vi "Client.vi"() -> ()   [LabVIEW 2020]
panel:
  in  "Tab Control":T1(tab)
  in  "Balcony Temperature Control":dbl
  in  "Bedroom 2 Temperature Control":dbl
  in  "Bedroom 1 Temperature Control":dbl
  in  "Kitchen Temperature Control":dbl
  in  "Master Bedroom Temperature Control":dbl
  in  "Time Control":dbl(knob) scale=0.0..24.0
  in  "Living Room Temperature Control":dbl
  in  "Light Rotation":bool
  in  "Balcony Alarm":bool
  in  "Bedroom 2 Alarm":bool
  in  "Bedroom 1 Alarm":bool
  in  "Kitchen Alarm":bool
  in  "Master Bedroom Alarm":bool
  in  "Automatic Curtain":bool
  in  "Living Room Alarm":bool
  in  "Curtains Master Button":bool
  in  "Doors Master Button":bool
  in  "Lights Master Button":bool
  in  "TV Brightness":dbl(knob) scale=1.0..6.0
  in  "Adaptive Brightness":bool
  in  "TV Volume":i32(knob) scale=0.0..100.0
  in  "TV Fast Forward Reverse":bool
  in  "TV Fast Forward":bool
  in  "TV Channel 2":bool
  in  "TV Channel 1":bool
  in  "TV Pause":bool
  in  "TV Play":bool
  in  "TV On/Off":bool
  in  "Living Room Curtain":bool
  in  "Living Room Light 1":bool
  in  "Living Room Light 2":bool
  in  "Living Room Light 1 Dim":bool
  in  "Living Room Light 2 Dim":bool
  in  "Living Room Door":bool
  in  "Master Bedroom AC":bool
  in  "Master Bedroom Curtain":bool
  in  "Master Bedroom Door":bool
  in  "Master Bedroom Light 2 Dim":bool
  in  "Master Bedroom Light 1 Dim":bool
  in  "Master Bedroom Light 2":bool
  in  "Master Bedroom Light 1":bool
  in  "Bedroom 1 Door":bool
  in  "Bedroom 1 Curtain":bool
  in  "Bedroom 1 Light 1 Dim":bool
  in  "Bedroom 1 Light 1":bool
  in  "Bedroom 2 Door":bool
  in  "Bedroom 2 Curtain":bool
  in  "Bedroom 2 Light 1 Dim":bool
  in  "Bedroom 2 Light 1":bool
  in  "Balcony Door 2":bool
  in  "Balcony Door 1":bool
  in  "Balcony Light 3 Dim":bool
  in  "Balcony Light 2 Dim":bool
  in  "Balcony Light 1 Dim":bool
  in  "Balcony Light 3":bool
  in  "Balcony Light 2":bool
  in  "Balcony Light 1":bool
  in  "Kitchen Door 2":bool
  in  "Kitchen Door 1":bool
  in  "Kitchen Light 1 Dim":bool
  in  "Kitchen Light 1":bool
  in  "stop":bool
  # "CLIENT"
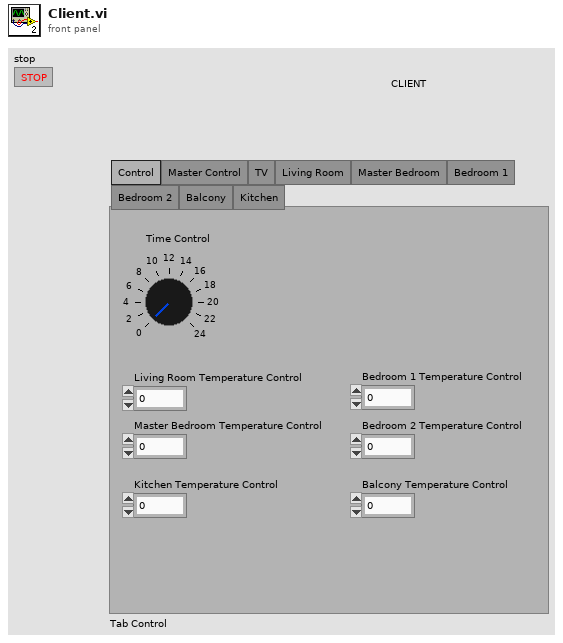
[diagram p1: front panel]
types:
  T1 = enum32{"Control", "Master Control", "TV", "Living Room", "Master Bedroom", "Bedroom 1", "Bedroom 2", "Balcony", "Kitchen"}
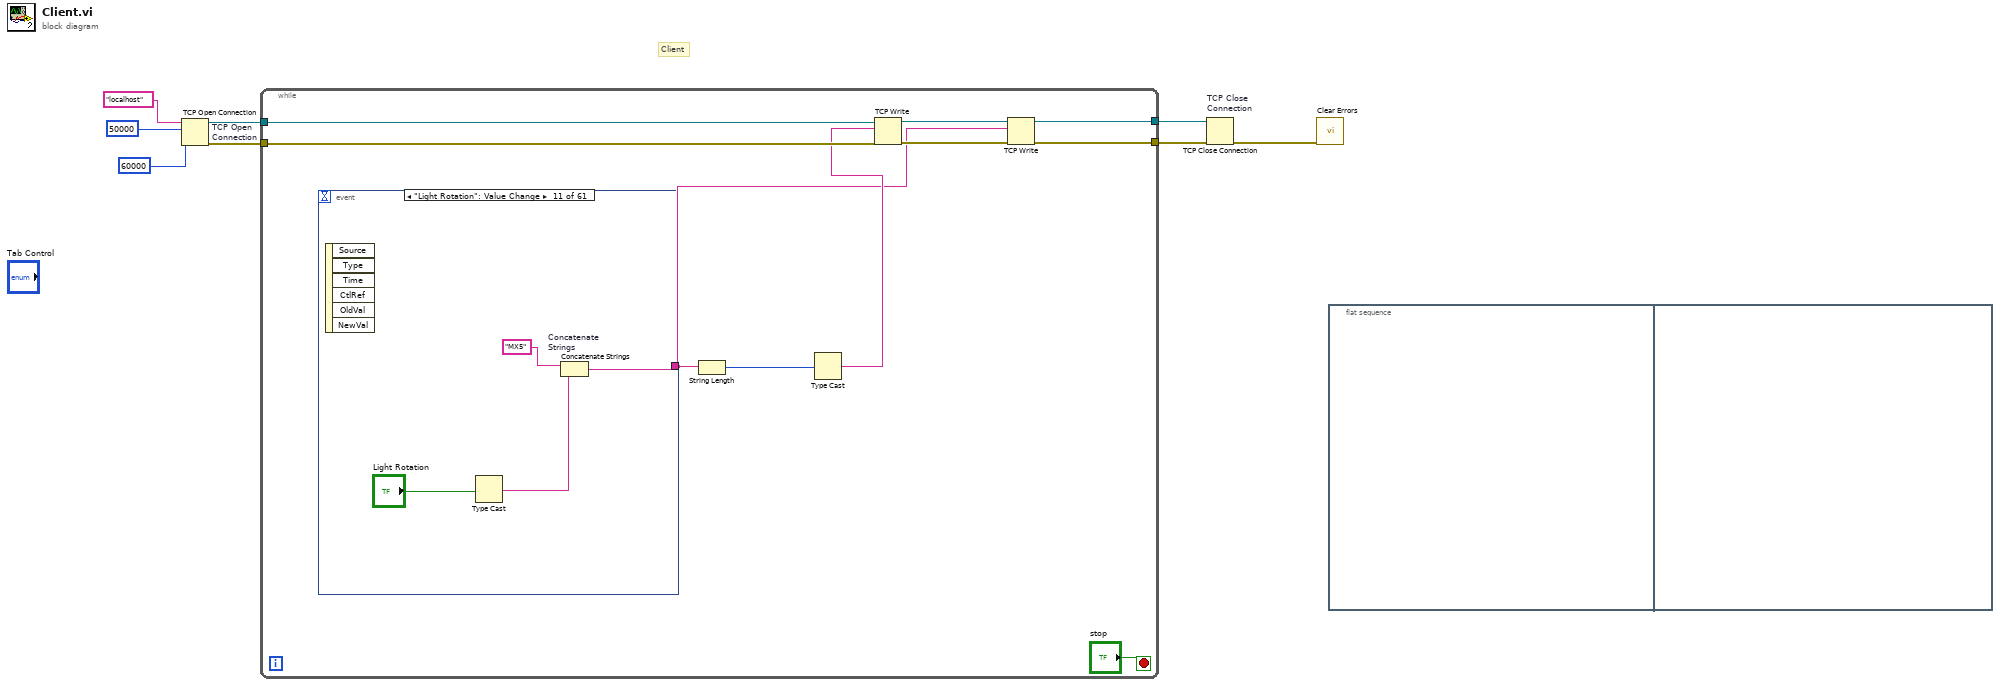
[diagram p0: block diagram]
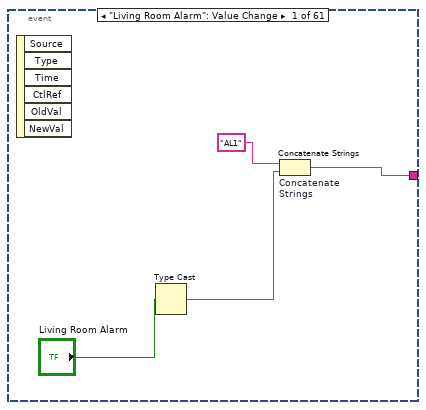
[diagram p2: hidden frame]
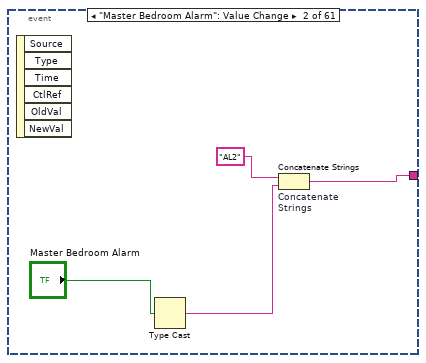
[diagram p3: hidden frame]
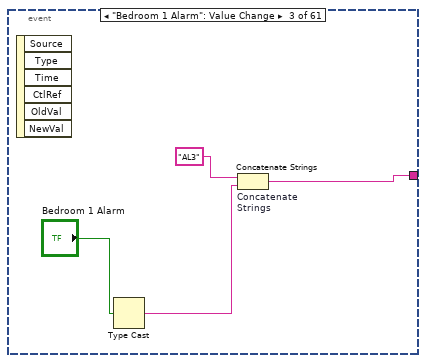
[diagram p4: hidden frame]
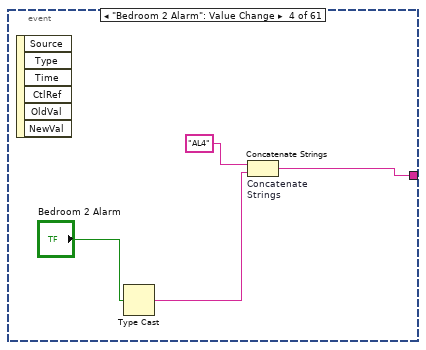
[diagram p5: hidden frame]
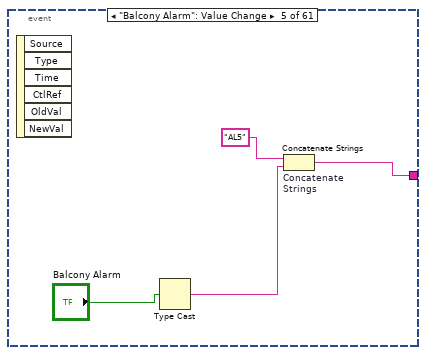
[diagram p6: hidden frame]
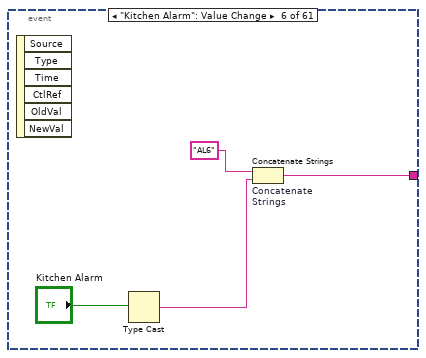
[diagram p7: hidden frame]
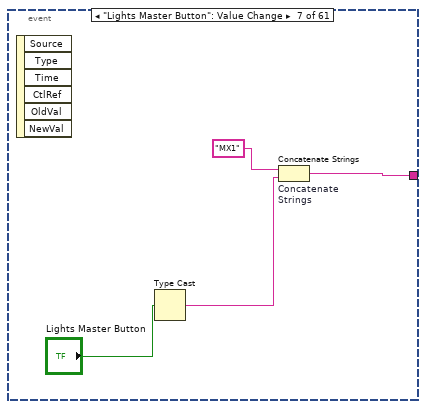
[diagram p8: hidden frame]
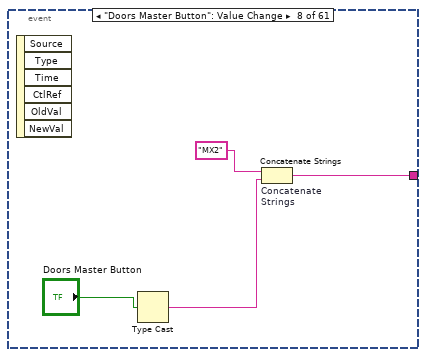
[diagram p9: hidden frame]
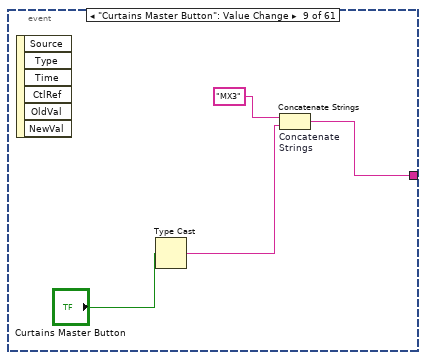
[diagram p10: hidden frame]
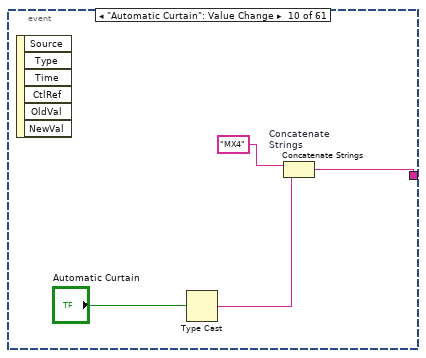
[diagram p11: hidden frame]
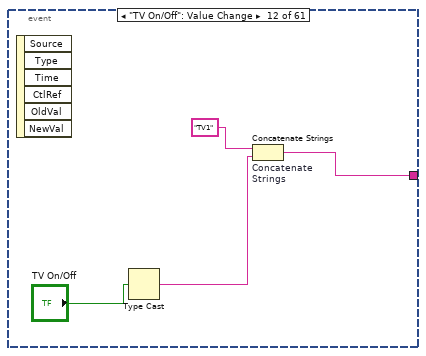
[diagram p12: hidden frame]
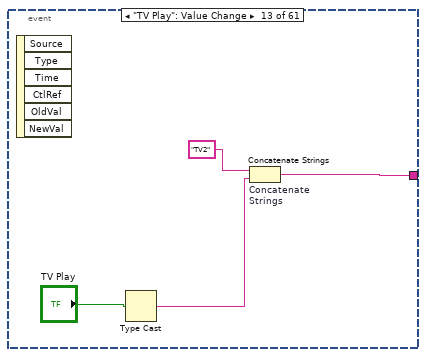
[diagram p13: hidden frame]
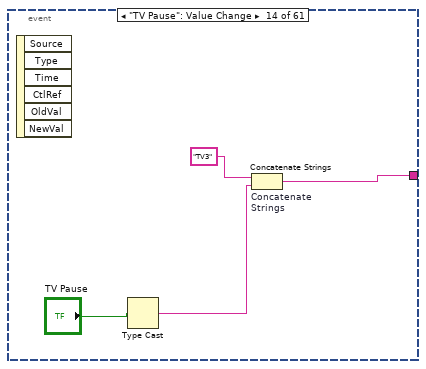
[diagram p14: hidden frame]
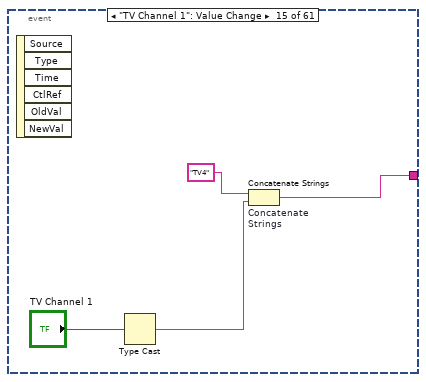
[diagram p15: hidden frame]
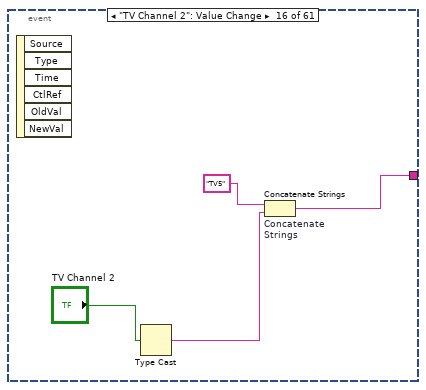
[diagram p16: hidden frame]
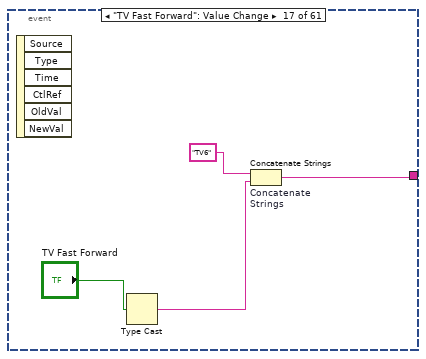
[diagram p17: hidden frame]
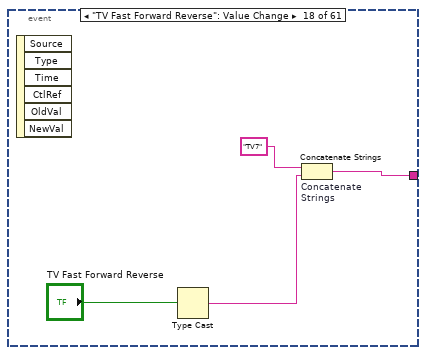
[diagram p18: hidden frame]
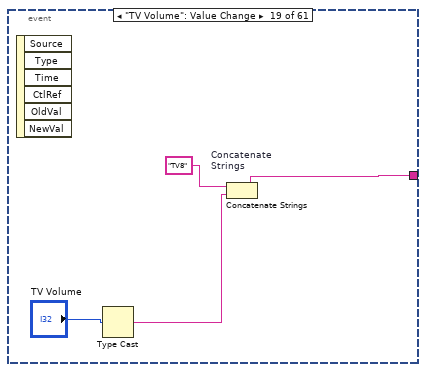
[diagram p19: hidden frame]
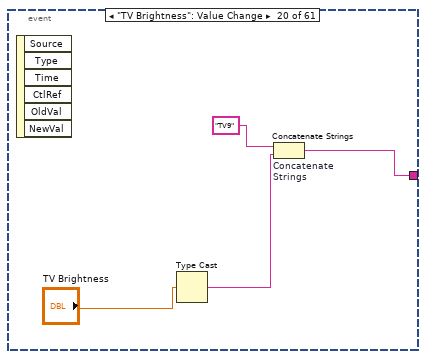
[diagram p20: hidden frame]
diagram:
  # "Client"
  n1 = TCP Open Connection "TCP Open \nConnection"(address="localhost", remote port or service name=u16 50000, timeout ms (60000)=60000) -> (connection ID=w5:refnum<k5>, error out=w3:errorcluster)  [unwired: 2 in]
  n2 = while {
    tunnel: w5 -> [w17]
    tunnel: [w15] -> w4
    tunnel: w3 -> [w14]
    tunnel: [w12] -> w2
    stop <- "stop" stop-if-true
    n3 = event shown="[10] \"Light Rotation\": Value Change" {
      selector: _ -> [_ _ _ _ _ _ _ _ _ _ _ _ _ _ _ _ _ _ _ _ _ _ _ _ _ _ _ _ _ _ _ _ _ _ _ _ _ _ _ _ _ _ _ _ _ _ _ _ _ _ _ _ _ _ _ _ _ _ _ _ _]
      dyn-events: _ -> [_ _ _ _ _ _ _ _ _ _ _ _ _ _ _ _ _ _ _ _ _ _ _ _ _ _ _ _ _ _ _ _ _ _ _ _ _ _ _ _ _ _ _ _ _ _ _ _ _ _ _ _ _ _ _ _ _ _ _ _ _]
      timeout: _ -> [_ _ _ _ _ _ _ _ _ _ _ _ _ _ _ _ _ _ _ _ _ _ _ _ _ _ _ _ _ _ _ _ _ _ _ _ _ _ _ _ _ _ _ _ _ _ _ _ _ _ _ _ _ _ _ _ _ _ _ _ _]
      tunnel: [w20 w24 w28 w32 w36 w40 w43 w48 w51 w55 w60 w63 w68 w72 w75 w80 w84 w87 w91 w96 w99 w105 w108 w112 w116 w120 w124 w127 w131 w136 w139 w144 w148 w152 w155 w160 w163 w168 w171 w176 w180 w183 w188 w192 w195 w199 w203 w208 w212 w216 w220 w224 w228 w232 w236 w240 w244 w248 w252 w256 w260] -> w9
      event "Living Room Alarm": Value Change {
        n4 = event-data() -> ()  [unwired: 1 in, 6 out]
        n5 = Type Cast(x="Living Room Alarm") -> (*(type *) &x=w22:string)  [unwired: 1 in]
        n6 = Concatenate Strings "Concatenate \nStrings"("AL1" ("string"), w22) -> (w20:string)
      }
      event "Master Bedroom Alarm": Value Change {
        n7 = event-data() -> ()  [unwired: 1 in, 6 out]
        n8 = Type Cast(x="Master Bedroom Alarm") -> (*(type *) &x=w26:string)  [unwired: 1 in]
        n9 = Concatenate Strings "Concatenate \nStrings"("AL2" ("string"), w26) -> (w24:string)
      }
      event "Bedroom 1 Alarm": Value Change {
        n10 = event-data() -> ()  [unwired: 1 in, 6 out]
        n11 = Type Cast(x="Bedroom 1 Alarm") -> (*(type *) &x=w30:string)  [unwired: 1 in]
        n12 = Concatenate Strings "Concatenate \nStrings"("AL3" ("string"), w30) -> (w28:string)
      }
      event "Bedroom 2 Alarm": Value Change {
        n13 = event-data() -> ()  [unwired: 1 in, 6 out]
        n14 = Type Cast(x="Bedroom 2 Alarm") -> (*(type *) &x=w34:string)  [unwired: 1 in]
        n15 = Concatenate Strings "Concatenate \nStrings"("AL4" ("string"), w34) -> (w32:string)
      }
      event "Balcony Alarm": Value Change {
        n16 = event-data() -> ()  [unwired: 1 in, 6 out]
        n17 = Type Cast(x="Balcony Alarm") -> (*(type *) &x=w38:string)  [unwired: 1 in]
        n18 = Concatenate Strings "Concatenate \nStrings"("AL5" ("string"), w38) -> (w36:string)
      }
      event "Kitchen Alarm": Value Change {
        n19 = event-data() -> ()  [unwired: 1 in, 6 out]
        n20 = Type Cast(x="Kitchen Alarm") -> (*(type *) &x=w42:string)  [unwired: 1 in]
        n21 = Concatenate Strings "Concatenate \nStrings"("AL6" ("string"), w42) -> (w40:string)
      }
      event "Lights Master Button": Value Change {
        n22 = event-data() -> ()  [unwired: 1 in, 6 out]
        n23 = Type Cast(x="Lights Master Button") -> (*(type *) &x=w45:string)  [unwired: 1 in]
        n24 = Concatenate Strings "Concatenate \nStrings"("MX1" ("string"), w45) -> (w43:string)
      }
      event "Doors Master Button": Value Change {
        n25 = event-data() -> ()  [unwired: 1 in, 6 out]
        n26 = Type Cast(x="Doors Master Button") -> (*(type *) &x=w50:string)  [unwired: 1 in]
        n27 = Concatenate Strings "Concatenate \nStrings"("MX2" ("string"), w50) -> (w48:string)
      }
      event "Curtains Master Button": Value Change {
        n28 = event-data() -> ()  [unwired: 1 in, 6 out]
        n29 = Type Cast(x="Curtains Master Button") -> (*(type *) &x=w54:string)  [unwired: 1 in]
        n30 = Concatenate Strings "Concatenate \nStrings"("MX3" ("string"), w54) -> (w51:string)
      }
      event "Automatic Curtain": Value Change {
        n31 = event-data() -> ()  [unwired: 1 in, 6 out]
        n32 = Type Cast(x="Automatic Curtain") -> (*(type *) &x=w57:string)  [unwired: 1 in]
        n33 = Concatenate Strings "Concatenate \nStrings"("MX4" ("string"), w57) -> (w55:string)
      }
      event "Light Rotation": Value Change {
        n34 = event-data() -> ()  [unwired: 1 in, 6 out]
        n35 = Type Cast(x="Light Rotation") -> (*(type *) &x=w62:string)  [unwired: 1 in]
        n36 = Concatenate Strings "Concatenate \nStrings"("MX5" ("string"), w62) -> (w60:string)
      }
      event "TV On/Off": Value Change {
        n37 = event-data() -> ()  [unwired: 1 in, 6 out]
        n38 = Type Cast(x="TV On/Off") -> (*(type *) &x=w66:string)  [unwired: 1 in]
        n39 = Concatenate Strings "Concatenate \nStrings"("TV1" ("string"), w66) -> (w63:string)
      }
      event "TV Play": Value Change {
        n40 = event-data() -> ()  [unwired: 1 in, 6 out]
        n41 = Type Cast(x="TV Play") -> (*(type *) &x=w70:string)  [unwired: 1 in]
        n42 = Concatenate Strings "Concatenate \nStrings"("TV2" ("string"), w70) -> (w68:string)
      }
      event "TV Pause": Value Change {
        n43 = event-data() -> ()  [unwired: 1 in, 6 out]
        n44 = Type Cast(x="TV Pause") -> (*(type *) &x=w74:string)  [unwired: 1 in]
        n45 = Concatenate Strings "Concatenate \nStrings"("TV3" ("string"), w74) -> (w72:string)
      }
      event "TV Channel 1": Value Change {
        n46 = event-data() -> ()  [unwired: 1 in, 6 out]
        n47 = Type Cast(x="TV Channel 1") -> (*(type *) &x=w78:string)  [unwired: 1 in]
        n48 = Concatenate Strings "Concatenate \nStrings"("TV4" ("string"), w78) -> (w75:string)
      }
      event "TV Channel 2": Value Change {
        n49 = event-data() -> ()  [unwired: 1 in, 6 out]
        n50 = Type Cast(x="TV Channel 2") -> (*(type *) &x=w82:string)  [unwired: 1 in]
        n51 = Concatenate Strings "Concatenate \nStrings"("TV5" ("string"), w82) -> (w80:string)
      }
      event "TV Fast Forward": Value Change {
        n52 = event-data() -> ()  [unwired: 1 in, 6 out]
        n53 = Type Cast(x="TV Fast Forward") -> (*(type *) &x=w86:string)  [unwired: 1 in]
        n54 = Concatenate Strings "Concatenate \nStrings"("TV6" ("string"), w86) -> (w84:string)
      }
      event "TV Fast Forward Reverse": Value Change {
        n55 = event-data() -> ()  [unwired: 1 in, 6 out]
        n56 = Type Cast(x="TV Fast Forward Reverse") -> (*(type *) &x=w90:string)  [unwired: 1 in]
        n57 = Concatenate Strings "Concatenate \nStrings"("TV7" ("string"), w90) -> (w87:string)
      }
      event "TV Volume": Value Change {
        n58 = event-data() -> ()  [unwired: 1 in, 6 out]
        n59 = Type Cast(x="TV Volume") -> (*(type *) &x=w94:string)  [unwired: 1 in]
        n60 = Concatenate Strings "Concatenate \nStrings"("TV8" ("string"), w94) -> (w91:string)
      }
      event "TV Brightness": Value Change {
        n61 = event-data() -> ()  [unwired: 1 in, 6 out]
        n62 = Type Cast(x="TV Brightness") -> (*(type *) &x=w98:string)  [unwired: 1 in]
        n63 = Concatenate Strings "Concatenate \nStrings"("TV9" ("string"), w98) -> (w96:string)
      }
      event "Adaptive Brightness": Value Change {
        n64 = event-data() -> ()  [unwired: 1 in, 6 out]
        n65 = Type Cast(x="Adaptive Brightness") -> (*(type *) &x=w102:string)  [unwired: 1 in]
        n66 = Concatenate Strings "Concatenate \nStrings"("TV10" ("string"), w102) -> (w99:string)
      }
      event "Living Room Temperature Control": Value Change {
        n67 = event-data() -> ()  [unwired: 1 in, 6 out]
        n68 = Type Cast(x="Living Room Temperature Control") -> (*(type *) &x=w104:string)  [unwired: 1 in]
        n69 = Concatenate Strings "Concatenate \nStrings"("HX1" ("string"), w104) -> (w105:string)
      }
      event "Master Bedroom Temperature Control": Value Change {
        n70 = event-data() -> ()  [unwired: 1 in, 6 out]
        n71 = Type Cast(x="Master Bedroom Temperature Control") -> (*(type *) &x=w110:string)  [unwired: 1 in]
        n72 = Concatenate Strings "Concatenate \nStrings"("HX3" ("string"), w110) -> (w108:string)
      }
      event "Bedroom 1 Temperature Control": Value Change {
        n73 = event-data() -> ()  [unwired: 1 in, 6 out]
        n74 = Type Cast(x="Bedroom 1 Temperature Control") -> (*(type *) &x=w113:string)  [unwired: 1 in]
        n75 = Concatenate Strings "Concatenate \nStrings"("HX4" ("string"), w113) -> (w112:string)
      }
      event "Bedroom 2 Temperature Control": Value Change {
        n76 = event-data() -> ()  [unwired: 1 in, 6 out]
        n77 = Type Cast(x="Bedroom 2 Temperature Control") -> (*(type *) &x=w118:string)  [unwired: 1 in]
        n78 = Concatenate Strings "Concatenate \nStrings"("HX5" ("string"), w118) -> (w116:string)
      }
      event "Balcony Temperature Control": Value Change {
        n79 = event-data() -> ()  [unwired: 1 in, 6 out]
        n80 = Type Cast(x="Balcony Temperature Control") -> (*(type *) &x=w122:string)  [unwired: 1 in]
        n81 = Concatenate Strings "Concatenate \nStrings"("HX6" ("string"), w122) -> (w120:string)
      }
      event "Kitchen Temperature Control": Value Change {
        n82 = event-data() -> ()  [unwired: 1 in, 6 out]
        n83 = Type Cast(x="Kitchen Temperature Control") -> (*(type *) &x=w125:string)  [unwired: 1 in]
        n84 = Concatenate Strings "Concatenate \nStrings"("HX7" ("string"), w125) -> (w124:string)
      }
      event "Time Control": Value Change {
        n85 = event-data() -> ()  [unwired: 1 in, 6 out]
        n86 = Type Cast(x="Time Control") -> (*(type *) &x=w129:string)  [unwired: 1 in]
        n87 = Concatenate Strings "Concatenate \nStrings"("HX2" ("string"), w129) -> (w127:string)
      }
      event "Living Room Light 1": Value Change {
        n88 = event-data() -> ()  [unwired: 1 in, 6 out]
        n89 = Type Cast(x="Living Room Light 1") -> (*(type *) &x=w134:string)  [unwired: 1 in]
        n90 = Concatenate Strings "Concatenate \nStrings"("LR1" ("string"), w134) -> (w131:string)
      }
      event "Living Room Light 2": Value Change {
        n91 = event-data() -> ()  [unwired: 1 in, 6 out]
        n92 = Type Cast(x="Living Room Light 2") -> (*(type *) &x=w138:string)  [unwired: 1 in]
        n93 = Concatenate Strings "Concatenate \nStrings"("LR2" ("string"), w138) -> (w136:string)
      }
      event "Living Room Light 1 Dim": Value Change {
        n94 = event-data() -> ()  [unwired: 1 in, 6 out]
        n95 = Type Cast(x="Living Room Light 1 Dim") -> (*(type *) &x=w142:string)  [unwired: 1 in]
        n96 = Concatenate Strings "Concatenate \nStrings"("LR3" ("string"), w142) -> (w139:string)
      }
      event "Living Room Light 2 Dim": Value Change {
        n97 = event-data() -> ()  [unwired: 1 in, 6 out]
        n98 = Type Cast(x="Living Room Light 2 Dim") -> (*(type *) &x=w146:string)  [unwired: 1 in]
        n99 = Concatenate Strings "Concatenate \nStrings"("LR4" ("string"), w146) -> (w144:string)
      }
      event "Living Room Curtain": Value Change {
        n100 = event-data() -> ()  [unwired: 1 in, 6 out]
        n101 = Type Cast(x="Living Room Curtain") -> (*(type *) &x=w150:string)  [unwired: 1 in]
        n102 = Concatenate Strings "Concatenate \nStrings"("LR5" ("string"), w150) -> (w148:string)
      }
      event "Living Room Door": Value Change {
        n103 = event-data() -> ()  [unwired: 1 in, 6 out]
        n104 = Type Cast(x="Living Room Door") -> (*(type *) &x=w154:string)  [unwired: 1 in]
        n105 = Concatenate Strings "Concatenate \nStrings"("LR6" ("string"), w154) -> (w152:string)
      }
      event "Master Bedroom Light 1": Value Change {
        n106 = event-data() -> ()  [unwired: 1 in, 6 out]
        n107 = Type Cast(x="Master Bedroom Light 1") -> (*(type *) &x=w158:string)  [unwired: 1 in]
        n108 = Concatenate Strings "Concatenate \nStrings"("MB1" ("string"), w158) -> (w155:string)
      }
      event "Master Bedroom Light 2": Value Change {
        n109 = event-data() -> ()  [unwired: 1 in, 6 out]
        n110 = Type Cast(x="Master Bedroom Light 2") -> (*(type *) &x=w162:string)  [unwired: 1 in]
        n111 = Concatenate Strings "Concatenate \nStrings"("MB2" ("string"), w162) -> (w160:string)
      }
      event "Master Bedroom Light 1 Dim": Value Change {
        n112 = event-data() -> ()  [unwired: 1 in, 6 out]
        n113 = Type Cast(x="Master Bedroom Light 1 Dim") -> (*(type *) &x=w166:string)  [unwired: 1 in]
        n114 = Concatenate Strings "Concatenate \nStrings"("MB3" ("string"), w166) -> (w163:string)
      }
      event "Master Bedroom Light 2 Dim": Value Change {
        n115 = event-data() -> ()  [unwired: 1 in, 6 out]
        n116 = Type Cast(x="Master Bedroom Light 2 Dim") -> (*(type *) &x=w170:string)  [unwired: 1 in]
        n117 = Concatenate Strings "Concatenate \nStrings"("MB4" ("string"), w170) -> (w168:string)
      }
      event "Master Bedroom Curtain": Value Change {
        n118 = event-data() -> ()  [unwired: 1 in, 6 out]
        n119 = Type Cast(x="Master Bedroom Curtain") -> (*(type *) &x=w174:string)  [unwired: 1 in]
        n120 = Concatenate Strings "Concatenate \nStrings"("MB5" ("string"), w174) -> (w171:string)
      }
      event "Master Bedroom Door": Value Change {
        n121 = event-data() -> ()  [unwired: 1 in, 6 out]
        n122 = Type Cast(x="Master Bedroom Door") -> (*(type *) &x=w178:string)  [unwired: 1 in]
        n123 = Concatenate Strings "Concatenate \nStrings"("MB6" ("string"), w178) -> (w176:string)
      }
      event "Master Bedroom AC": Value Change {
        n124 = event-data() -> ()  [unwired: 1 in, 6 out]
        n125 = Type Cast(x="Master Bedroom AC") -> (*(type *) &x=w182:string)  [unwired: 1 in]
        n126 = Concatenate Strings "Concatenate \nStrings"("MB7" ("string"), w182) -> (w180:string)
      }
      event "Bedroom 1 Light 1": Value Change {
        n127 = event-data() -> ()  [unwired: 1 in, 6 out]
        n128 = Type Cast(x="Bedroom 1 Light 1") -> (*(type *) &x=w186:string)  [unwired: 1 in]
        n129 = Concatenate Strings "Concatenate \nStrings"("B11" ("string"), w186) -> (w183:string)
      }
      event "Bedroom 1 Light 1 Dim": Value Change {
        n130 = event-data() -> ()  [unwired: 1 in, 6 out]
        n131 = Type Cast(x="Bedroom 1 Light 1 Dim") -> (*(type *) &x=w190:string)  [unwired: 1 in]
        n132 = Concatenate Strings "Concatenate \nStrings"("B12" ("string"), w190) -> (w188:string)
      }
      event "Bedroom 1 Curtain": Value Change {
        n133 = event-data() -> ()  [unwired: 1 in, 6 out]
        n134 = Type Cast(x="Bedroom 1 Curtain") -> (*(type *) &x=w194:string)  [unwired: 1 in]
        n135 = Concatenate Strings "Concatenate \nStrings"("B13" ("string"), w194) -> (w192:string)
      }
      event "Bedroom 1 Door": Value Change {
        n136 = event-data() -> ()  [unwired: 1 in, 6 out]
        n137 = Type Cast(x="Bedroom 1 Door") -> (*(type *) &x=w198:string)  [unwired: 1 in]
        n138 = Concatenate Strings "Concatenate \nStrings"("B14" ("string"), w198) -> (w195:string)
      }
      event "Bedroom 2 Light 1": Value Change {
        n139 = event-data() -> ()  [unwired: 1 in, 6 out]
        n140 = Type Cast(x="Bedroom 2 Light 1") -> (*(type *) &x=w202:string)  [unwired: 1 in]
        n141 = Concatenate Strings "Concatenate \nStrings"("B21" ("string"), w202) -> (w199:string)
      }
      event "Bedroom 2 Light 1 Dim": Value Change {
        n142 = event-data() -> ()  [unwired: 1 in, 6 out]
        n143 = Type Cast(x="Bedroom 2 Light 1 Dim") -> (*(type *) &x=w206:string)  [unwired: 1 in]
        n144 = Concatenate Strings "Concatenate \nStrings"("B22" ("string"), w206) -> (w203:string)
      }
      event "Bedroom 2 Curtain": Value Change {
        n145 = event-data() -> ()  [unwired: 1 in, 6 out]
        n146 = Type Cast(x="Bedroom 2 Curtain") -> (*(type *) &x=w210:string)  [unwired: 1 in]
        n147 = Concatenate Strings "Concatenate \nStrings"("B23" ("string"), w210) -> (w208:string)
      }
      event "Bedroom 2 Door": Value Change {
        n148 = event-data() -> ()  [unwired: 1 in, 6 out]
        n149 = Type Cast(x="Bedroom 2 Door") -> (*(type *) &x=w214:string)  [unwired: 1 in]
        n150 = Concatenate Strings "Concatenate \nStrings"("B24" ("string"), w214) -> (w212:string)
      }
      event "Balcony Light 1": Value Change {
        n151 = event-data() -> ()  [unwired: 1 in, 6 out]
        n152 = Type Cast(x="Balcony Light 1") -> (*(type *) &x=w218:string)  [unwired: 1 in]
        n153 = Concatenate Strings "Concatenate \nStrings"("BA1" ("string"), w218) -> (w216:string)
      }
      event "Balcony Light 2": Value Change {
        n154 = event-data() -> ()  [unwired: 1 in, 6 out]
        n155 = Type Cast(x="Balcony Light 2") -> (*(type *) &x=w222:string)  [unwired: 1 in]
        n156 = Concatenate Strings "Concatenate \nStrings"("BA2" ("string"), w222) -> (w220:string)
      }
      event "Balcony Light 3": Value Change {
        n157 = event-data() -> ()  [unwired: 1 in, 6 out]
        n158 = Type Cast(x="Balcony Light 3") -> (*(type *) &x=w226:string)  [unwired: 1 in]
        n159 = Concatenate Strings "Concatenate \nStrings"("BA3" ("string"), w226) -> (w224:string)
      }
      event "Balcony Light 1 Dim": Value Change {
        n160 = event-data() -> ()  [unwired: 1 in, 6 out]
        n161 = Type Cast(x="Balcony Light 1 Dim") -> (*(type *) &x=w230:string)  [unwired: 1 in]
        n162 = Concatenate Strings "Concatenate \nStrings"("BA4" ("string"), w230) -> (w228:string)
      }
      event "Balcony Light 2 Dim": Value Change {
        n163 = event-data() -> ()  [unwired: 1 in, 6 out]
        n164 = Type Cast(x="Balcony Light 2 Dim") -> (*(type *) &x=w234:string)  [unwired: 1 in]
        n165 = Concatenate Strings "Concatenate \nStrings"("BA5" ("string"), w234) -> (w232:string)
      }
      event "Balcony Light 3 Dim": Value Change {
        n166 = event-data() -> ()  [unwired: 1 in, 6 out]
        n167 = Type Cast(x="Balcony Light 3 Dim") -> (*(type *) &x=w238:string)  [unwired: 1 in]
        n168 = Concatenate Strings "Concatenate \nStrings"("BA6" ("string"), w238) -> (w236:string)
      }
      event "Balcony Door 1": Value Change {
        n169 = event-data() -> ()  [unwired: 1 in, 6 out]
        n170 = Type Cast(x="Balcony Door 1") -> (*(type *) &x=w242:string)  [unwired: 1 in]
        n171 = Concatenate Strings "Concatenate \nStrings"("BA7" ("string"), w242) -> (w240:string)
      }
      event "Balcony Door 2": Value Change {
        n172 = event-data() -> ()  [unwired: 1 in, 6 out]
        n173 = Type Cast(x="Balcony Door 2") -> (*(type *) &x=w246:string)  [unwired: 1 in]
        n174 = Concatenate Strings "Concatenate \nStrings"("BA8" ("string"), w246) -> (w244:string)
      }
      event "Kitchen Light 1": Value Change {
        n175 = event-data() -> ()  [unwired: 1 in, 6 out]
        n176 = Type Cast(x="Kitchen Light 1") -> (*(type *) &x=w250:string)  [unwired: 1 in]
        n177 = Concatenate Strings "Concatenate \nStrings"("KI1" ("string"), w250) -> (w248:string)
      }
      event "Kitchen Light 1 Dim": Value Change {
        n178 = event-data() -> ()  [unwired: 1 in, 6 out]
        n179 = Type Cast(x="Kitchen Light 1 Dim") -> (*(type *) &x=w254:string)  [unwired: 1 in]
        n180 = Concatenate Strings "Concatenate \nStrings"("KI2" ("string"), w254) -> (w252:string)
      }
      event "Kitchen Door 1": Value Change {
        n181 = event-data() -> ()  [unwired: 1 in, 6 out]
        n182 = Type Cast(x="Kitchen Door 1") -> (*(type *) &x=w258:string)  [unwired: 1 in]
        n183 = Concatenate Strings "Concatenate \nStrings"("KI3" ("string"), w258) -> (w256:string)
      }
      event "Kitchen Door 2": Value Change {
        n184 = event-data() -> ()  [unwired: 1 in, 6 out]
        n185 = Type Cast(x="Kitchen Door 2") -> (*(type *) &x=w262:string)  [unwired: 1 in]
        n186 = Concatenate Strings "Concatenate \nStrings"("KI4" ("string"), w262) -> (w260:string)
      }
    }
    n187 = String Length(string=w9) -> (length=w11:i32)
    n188 = Type Cast(x=w11) -> (*(type *) &x=w10:string)  [unwired: 1 in]
    n189 = TCP Write(connection ID=w17, data in=w10, error in (no error)=w14) -> (connection ID out=w16:refnum<k5>, error out=w13:errorcluster)  [unwired: 1 in, 1 out]
    n190 = TCP Write(connection ID=w16, data in=w9, error in (no error)=w13) -> (connection ID out=w15:refnum<k5>, error out=w12:errorcluster)  [unwired: 1 in, 1 out]
  }
  n191 = TCP Close Connection "TCP Close \nConnection"(connection ID=w4, error in (no error)=w2) -> (error out=w1:errorcluster)  [unwired: 1 in, 1 out]
  n192 = call <vilib>:"Clear Errors.vi"("error in (no error)"=w1) -> ()  [unwired: 5 in, 2 out]
  n193 = flat-sequence {
    frame #0 {
    }
    frame #1 {
    }
  }
